vi "Tacking Helper - Arm Lengths.vi"(6 "Bounding box\nside length (m?)":dbl, 9 "Second Angle":dbl, 10 "Starting Angle":dbl, 11 "Angle from boat\nto waypoint":dbl) -> (2 "Second\nArm Length":dbl, 3 "Starting\nArm Length":dbl)   [LabVIEW 2011]
doc: "This vi takes the 'boat to waypoint' angle and gets the absolute angle difference between each tack angle and the greater angle. By using the triangle formed by the tack path and the bounding box, we can get the starting arm length and secondary arm length."
uses:
  <vilib>/Analysis/coordinate.llb/Angle Units.ctl
  <vilib>/Analysis/coordinate.llb/Absolute Angle Difference (scalar).vi
  <vilib>/Analysis/coordinate.llb/Wrap Angle (scalar).vi
  <vilib>/Analysis/coordinate.llb/Set Angle Unit.vi
  <vilib>/Analysis/NI_AAL_Angle.lvlib
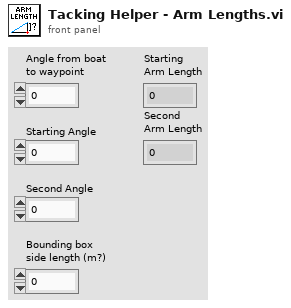
[diagram p1: front panel]
types:
  T1 = typedef "NI_AAL_Angle.lvlib/Angle Units.ctl" = i32
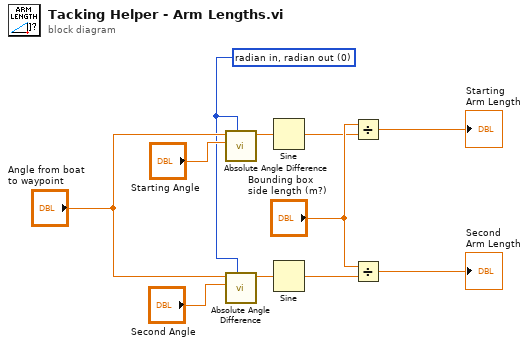
[diagram p0: block diagram]
diagram:
  w5 = T1 0 items=["radian in, radian out", "radian in, degree out", "degree in, degree out", "degree in, radian out"] ("angle units")
  n1 = call-poly <vilib>:"Absolute Angle Difference.vi"("angle units"=w5, "angle 2"="Starting Angle", "angle 1"="Angle from boat\nto waypoint") -> ("absolute angle difference"=w1:dbl)  [unwired: 7 in, 1 out]
  n2 = call-poly <vilib>:"Absolute Angle Difference.vi"("angle units"=w5, "angle 2"="Second Angle", "angle 1"="Angle from boat\nto waypoint") -> ("absolute angle difference"=w3:dbl)  [unwired: 7 in, 1 out]
  n3 = Sine(x=w1) -> (sin(x)=w2:dbl)
  n4 = Sine(x=w3) -> (sin(x)=w4:dbl)
  n5 = Divide(x="Bounding box\nside length (m?)", y=w2) -> (x/y=→"Starting\nArm Length":dbl)
  n6 = Divide(x="Bounding box\nside length (m?)", y=w4) -> (x/y=→"Second\nArm Length":dbl)
